vi "Initialise.vi"(10 "Diffuse Colour":refnum<vi>, 11 "Scene":refnum<vi>) -> (2 "Light Direction":T1, 3 "Core Data out":T2)   [LabVIEW 2022 SP3, in "Application.lvlib"]
uses:
  Application.lvlib
  Core Data.ctl
  Scene/Scene.lvclass
  Libraries/3D/Transform.ctl
  Libraries/3D/Vector 3D.ctl
  Libraries/Raster/Screen Dimensions.ctl
  Libraries/Raster/Raster.lvlib
  Libraries/3D/3D.lvlib
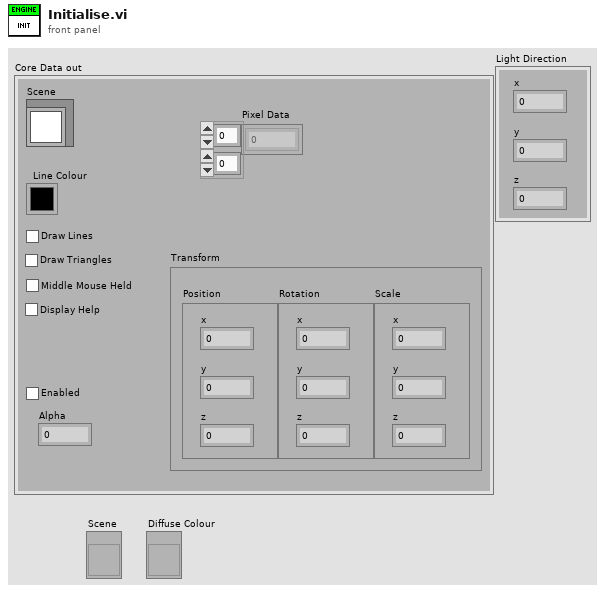
[diagram p1: front panel]
types:
  T1 = typedef "3D.lvlib/Vector 3D.ctl" = cluster{"x":sgl, "y":sgl, "z":sgl}
  T2 = typedef "Application.lvlib/Core Data.ctl" = cluster{"Line Colour":u32, "Draw Lines":bool, "Draw Triangles":bool, "Pixel Data":u32[][], "Middle Mouse Held":bool, "Scene":refnum<class "Scene.lvclass">, "Display Help":bool, "Transform":T3, "Enabled":bool, "Alpha":dbl}
  T3 = typedef "3D.lvlib/Transform.ctl" = cluster{"Position":T1, "Rotation":T1, "Scale":T1}
  T4 = typedef "Raster.lvlib/Screen Dimensions.ctl" = cluster{"Width":u32, "Height":u32}
  T5 = enum32{"invalid app kind", "Development System", "Run Time System", "Student Edition", "Embedded LabVIEW", "Evaluation", "Custom"}
  T6 = typedef "3D.lvlib/Object.ctl" = cluster{"Triangles":T7[], "Diffuse Colour":u32, "Transform":T3, "Name":string, "Enabled":bool, "Alpha":dbl}
  T7 = typedef "3D.lvlib/Triangle 3D.ctl" = cluster{"Point 1":T1, "Point 2":T1, "Point 3":T1}
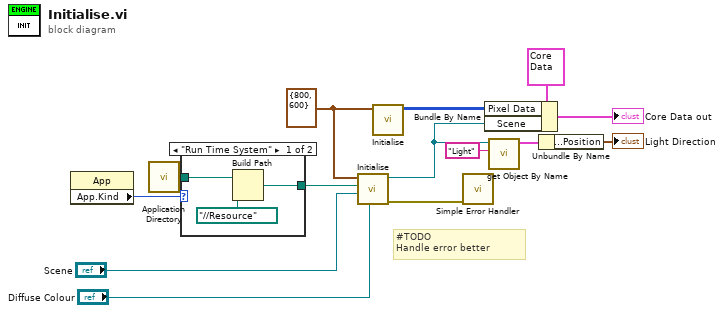
[diagram p0: block diagram]
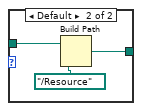
[diagram p2: hidden frame]
diagram:
  w7 = T4 {"Width"=800, "Height"=600} ("Screen Dimensions")
  # "#TODO\nHandle error better"
  n1 = property class="App"() -> ("App.Kind"=w10:T5)  [unwired: 2 in, 2 out]
  n2 = call <vilib>:"Application Directory.vi"() -> ("Application Directory"=w8:path)
  n3 = case shown="\"Run Time System\"" w10 {
    tunnel: [w17 w20] -> w9
    tunnel: w8 -> [w15 w18]
    frame "Run Time System" {
      n4 = Build Path(base path=w15, name or relative path=path "../../Resource") -> (appended path=w17:path)
    }
    frame Default {
      n5 = Build Path(base path=w18, name or relative path=path "../Resource") -> (appended path=w20:path)
    }
  }
  n6 = call "Initialise.vi"("Diffuse Colour"="Diffuse Colour", "Scene"="Scene", "Resource Directory"=w9, "Screen Dimensions"=w7) -> ("error out"=w11:errorcluster, "Scene out"=w4:refnum<class "Scene.lvclass">)  [unwired: 6 in]
  n7 = call "Initialise.vi"("Screen Dimensions"=w7) -> ("Pixel Data out"=w12:u32[][])  [unwired: 10 in]
  n8 = call <vilib>:"Simple Error Handler.vi"("error in (no error)"=w11) -> ()  [unwired: 4 in, 5 out]
  n9 = Bundle By Name(cluster=T2 {"Line Colour"=4375295, "Draw Lines"=FALSE, "Draw Triangles"=FALSE, "Pixel Data"=[], "Middle Mouse Held"=FALSE, "Scene"=refnum, "Display Help"=FALSE, "Transform"={"Position"={"x"=0.0, "y"=0.0, "z"=0.0}, "Rotation"={"x"=0.0, "y"=0.0, "z"=0.0}, "Scale"={"x"=0.0, "y"=0.0, "z"=0.0}}, "Enabled"=FALSE, "Alpha"=0.0} ("Core Data"), "Pixel Data"=w12, "Scene"=w4) -> (→"Core Data out":T2)
  n10 = call "get Object By Name.vi"("Name"="Light", "Scene in"=w4) -> ("Object"=w2:T6)  [unwired: 9 in]
  n11 = Unbundle By Name(w2) -> ("Transform.Position"=→"Light Direction":T1)
